vi "Update Status from Benchmarks.vi"(9 "CIFCorePlugin in":refnum<class "CIFCorePlugin.lvclass">) -> (1 "CIFCorePlugin out":refnum<class "CIFCorePlugin.lvclass">)   [LabVIEW 2021, in "CIFCorePlugin.lvclass"]
uses:
  CIFCorePlugin.lvclass
  CIFCorePlugin.lvclass/CIFCorePlugin.ctl
  <vilib>/CIF Foundation/CIF Utilities/Statistics/I64/Stats_I64_CIF_U.lvclass/Stats_I64_CIF_U.ctl
  <vilib>/CIF Foundation/CIF Utilities/Statistics/I64/Stats_I64_CIF_U.lvclass
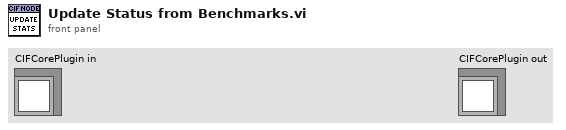
[diagram p1: front panel]
types:
  T1 = typedef "CIFCoreCommon.lvlib/Timing Statistics.ctl" = cluster{"Period":T2, "Wake Error":T2, "Execute":T2, "Housekeep":T2, "Idle":T2, "Cleanup":T2, "Custom 1 (custom units)":T2, "Custom 2 (custom units)":T2}
  T2 = typedef "CIFCoreCommon.lvlib/Timing Stats Base.ctl" = cluster{"Max":i64, "Avg":dbl, "Min":i64}
  T3 = typedef "CIFCoreCommon.lvlib/FIFO Statistics.ctl" = cluster{"From T0":T2, "From Previous Plugin":T2, "Output Error":T2}
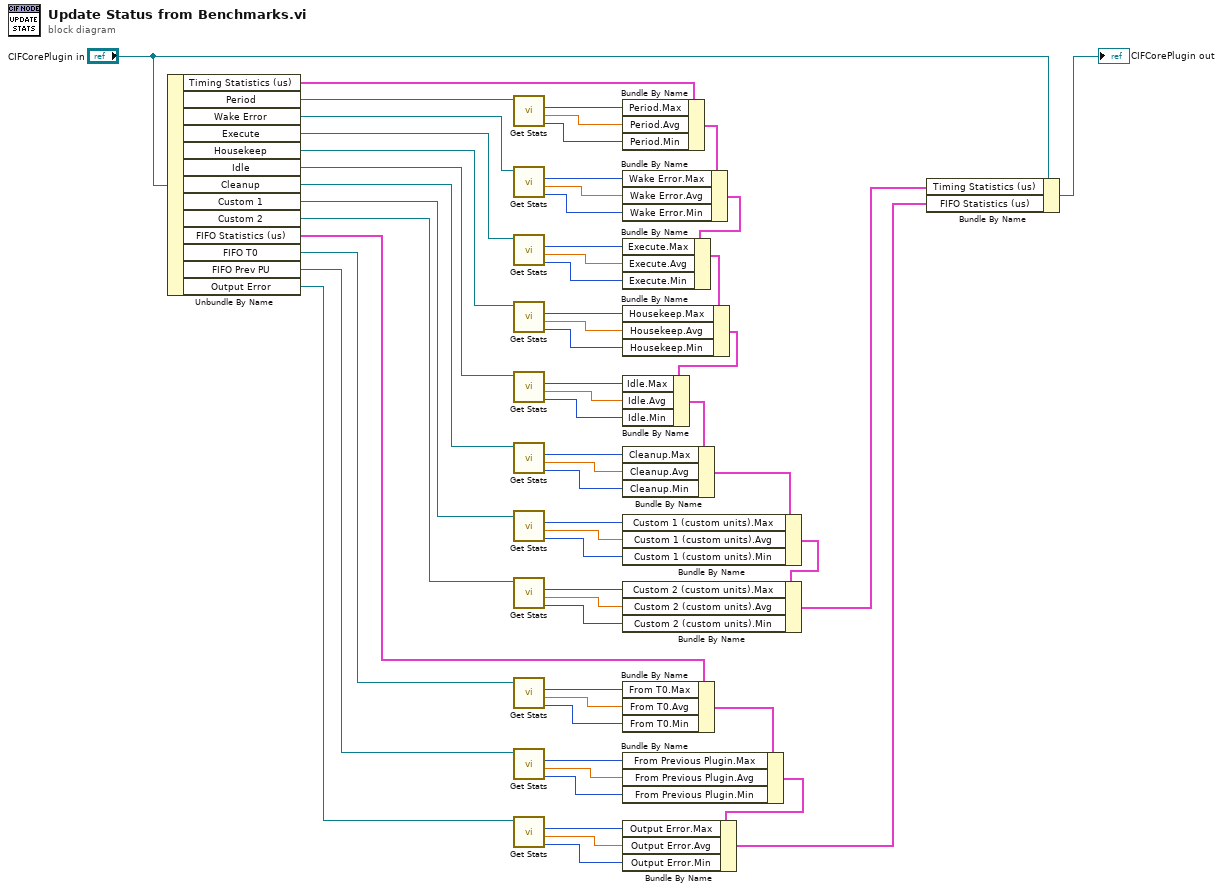
[diagram p0: block diagram]
diagram:
  n1 = Unbundle By Name("CIFCorePlugin in") -> ("Timing Statistics (us)"=w57:T1, "Period"=w13:refnum<class "Stats_I64_CIF_U.lvclass">, "Wake Error"=w12:refnum<class "Stats_I64_CIF_U.lvclass">, "Execute"=w11:refnum<class "Stats_I64_CIF_U.lvclass">, "Housekeep"=w10:refnum<class "Stats_I64_CIF_U.lvclass">, "Idle"=w9:refnum<class "Stats_I64_CIF_U.lvclass">, "Cleanup"=w8:refnum<class "Stats_I64_CIF_U.lvclass">, "Custom 1"=w7:refnum<class "Stats_I64_CIF_U.lvclass">, "Custom 2"=w6:refnum<class "Stats_I64_CIF_U.lvclass">, "FIFO Statistics (us)"=w2:T3, "FIFO T0"=w3:refnum<class "Stats_I64_CIF_U.lvclass">, "FIFO Prev PU"=w5:refnum<class "Stats_I64_CIF_U.lvclass">, "Output Error"=w4:refnum<class "Stats_I64_CIF_U.lvclass">)
  n2 = call <vilib>:"Get Stats.vi"("Stats_I64_CIF_U in"=w13) -> ("Min"=w55:i64, "Average"=w54:dbl, "Max"=w53:i64)  [unwired: 6 in, 2 out]
  n3 = call <vilib>:"Get Stats.vi"("Stats_I64_CIF_U in"=w12) -> ("Min"=w50:i64, "Average"=w51:dbl, "Max"=w52:i64)  [unwired: 6 in, 2 out]
  n4 = call <vilib>:"Get Stats.vi"("Stats_I64_CIF_U in"=w11) -> ("Min"=w49:i64, "Average"=w48:dbl, "Max"=w47:i64)  [unwired: 6 in, 2 out]
  n5 = call <vilib>:"Get Stats.vi"("Stats_I64_CIF_U in"=w10) -> ("Min"=w44:i64, "Average"=w45:dbl, "Max"=w46:i64)  [unwired: 6 in, 2 out]
  n6 = call <vilib>:"Get Stats.vi"("Stats_I64_CIF_U in"=w9) -> ("Min"=w26:i64, "Average"=w27:dbl, "Max"=w28:i64)  [unwired: 6 in, 2 out]
  n7 = call <vilib>:"Get Stats.vi"("Stats_I64_CIF_U in"=w8) -> ("Min"=w31:i64, "Average"=w30:dbl, "Max"=w29:i64)  [unwired: 6 in, 2 out]
  n8 = call <vilib>:"Get Stats.vi"("Stats_I64_CIF_U in"=w7) -> ("Min"=w32:i64, "Average"=w33:dbl, "Max"=w34:i64)  [unwired: 6 in, 2 out]
  n9 = call <vilib>:"Get Stats.vi"("Stats_I64_CIF_U in"=w6) -> ("Min"=w37:i64, "Average"=w36:dbl, "Max"=w35:i64)  [unwired: 6 in, 2 out]
  n10 = call <vilib>:"Get Stats.vi"("Stats_I64_CIF_U in"=w3) -> ("Min"=w14:i64, "Average"=w15:dbl, "Max"=w16:i64)  [unwired: 6 in, 2 out]
  n11 = call <vilib>:"Get Stats.vi"("Stats_I64_CIF_U in"=w5) -> ("Min"=w19:i64, "Average"=w18:dbl, "Max"=w17:i64)  [unwired: 6 in, 2 out]
  n12 = call <vilib>:"Get Stats.vi"("Stats_I64_CIF_U in"=w4) -> ("Min"=w20:i64, "Average"=w21:dbl, "Max"=w22:i64)  [unwired: 6 in, 2 out]
  n13 = Bundle By Name(cluster=w57, "Period.Max"=w53, "Period.Avg"=w54, "Period.Min"=w55) -> (w43:T1)
  n14 = Bundle By Name(cluster=w43, "Wake Error.Max"=w52, "Wake Error.Avg"=w51, "Wake Error.Min"=w50) -> (w42:T1)
  n15 = Bundle By Name(cluster=w42, "Execute.Max"=w47, "Execute.Avg"=w48, "Execute.Min"=w49) -> (w41:T1)
  n16 = Bundle By Name(cluster=w41, "Housekeep.Max"=w46, "Housekeep.Avg"=w45, "Housekeep.Min"=w44) -> (w25:T1)
  n17 = Bundle By Name(cluster=w25, "Idle.Max"=w28, "Idle.Avg"=w27, "Idle.Min"=w26) -> (w38:T1)
  n18 = Bundle By Name(cluster=w38, "Cleanup.Max"=w29, "Cleanup.Avg"=w30, "Cleanup.Min"=w31) -> (w39:T1)
  n19 = Bundle By Name(cluster=w39, "Custom 1 (custom units).Max"=w34, "Custom 1 (custom units).Avg"=w33, "Custom 1 (custom units).Min"=w32) -> (w40:T1)
  n20 = Bundle By Name(cluster=w40, "Custom 2 (custom units).Max"=w35, "Custom 2 (custom units).Avg"=w36, "Custom 2 (custom units).Min"=w37) -> (w56:T1)
  n21 = Bundle By Name(cluster=w2, "From T0.Max"=w16, "From T0.Avg"=w15, "From T0.Min"=w14) -> (w23:T3)
  n22 = Bundle By Name(cluster=w23, "From Previous Plugin.Max"=w17, "From Previous Plugin.Avg"=w18, "From Previous Plugin.Min"=w19) -> (w24:T3)
  n23 = Bundle By Name(cluster=w24, "Output Error.Max"=w22, "Output Error.Avg"=w21, "Output Error.Min"=w20) -> (w1:T3)
  n24 = Bundle By Name(cluster="CIFCorePlugin in", "Timing Statistics (us)"=w56, "FIFO Statistics (us)"=w1) -> (→"CIFCorePlugin out":refnum<class "CIFCorePlugin.lvclass">)
